vi "Read As ByteArray.vi"(8 "error in (no error)":errorcluster, 11 "HttpContent in":refnum<class "HttpContent.lvclass">) -> (0 "error out":errorcluster, 1 "Content":u8[](array[numeric]), 3 "HttpContent out":refnum<class "HttpContent.lvclass">)   [LabVIEW 2018, in "HttpClient_NET.lvlib" / "HttpContent.lvclass"]
uses:
  HttpContent.lvclass
  HttpContent.lvclass/HttpContent.ctl
  System.Net.Http
  Accessors/Read NET_HttpContent.vi
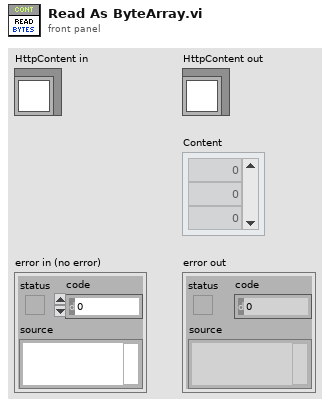
[diagram p1: front panel]
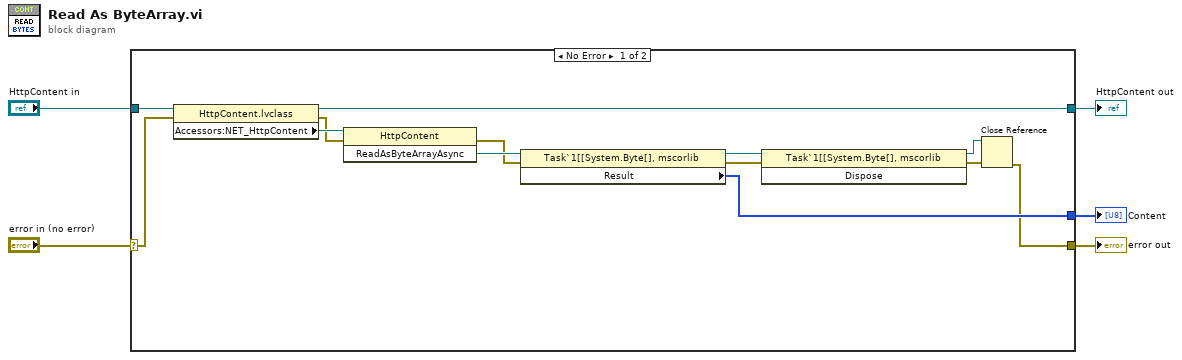
[diagram p0: block diagram]
diagram:
  n1 = case shown="No Error" "error in (no error)" {
    selector: "error in (no error)" -> [w7 w20]
    tunnel: [w6 w20] -> w4
    tunnel: [w17 w19] -> w2
    tunnel: "HttpContent in" -> [w18 w19]
    tunnel: [w14 _] -> w1
    frame No Error {
      n2 = property class="HttpContent.lvclass"(reference=w18, error in=w7) -> (reference out=w17:refnum<class "HttpContent.lvclass">, error out=w13:errorcluster, "Accessors:NET_HttpContent"=w16:refnum<k24>)
      n3 = invoke class="HttpContent" method="ReadAsByteArrayAsync"(reference=w16, error in=w13) -> (error out=w12:errorcluster, "ReadAsByteArrayAsync"=w15:refnum<k24>)  [unwired: 1 in, 1 out]
      n4 = property class="Task`1[[System.Byte[], mscorlib"(reference=w15, error in=w12) -> (reference out=w11:refnum<k24>, error out=w10:errorcluster, "Result"=w14:u8[])
      n5 = invoke class="Task`1[[System.Byte[], mscorlib" method="Dispose"(reference=w11, error in=w10) -> (reference out=w8:refnum<k24>, error out=w9:errorcluster)  [unwired: 1 in, 1 out]
      n6 = Close Reference(reference=w8, error in (no error)=w9) -> (error out=w6:errorcluster)
    }
    frame Error {
    }
  }
  "error out" <- w4
  "HttpContent out" <- w2
  "Content" <- w1
